vi "Close camera.vi"(8 "error in (no error)":errorcluster, 11 "camera handle in":i16) -> (0 "error out":errorcluster)   [LabVIEW 2012]
uses:
  Visual Studio/Cascade wrapper/Release/Cascade wrapper.dll
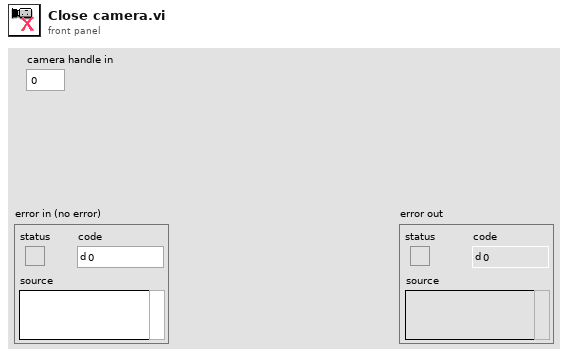
[diagram p1: front panel]
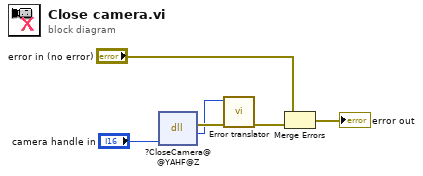
[diagram p0: block diagram]
diagram:
  n1 = dll-call lib="C:/moroder/Cascade wrapper/Visual Studio/Cascade wrapper/Release/Cascade wrapper.dll" fn="?CloseCamera@@YAHF@Z"("camera handle"="camera handle in") -> (error out=w4:errorcluster, "error"=w3:i32)  [unwired: 4 in, 1 out]
  n2 = call "Error translator.vi"("error in (no error)"=w4, "error code"=w3) -> ("error out"=w5:errorcluster)  [unwired: 9 in]
  n3 = Merge Errors("error in (no error)", w5) -> (→"error out":errorcluster)
